vi "AbortAllMovements.vi"(8 "error in (no error)":errorcluster, 11 "CS++Motor in":refnum<class "CS++Motor.lvclass">) -> (0 "error out":errorcluster, 3 "CS++Motor out":refnum<class "CS++Motor.lvclass">)   [LabVIEW 2015, in "CS++Motor.lvlib" / "CS++Motor.lvclass"]
doc: "Stops the movement of all axes immeadiately."
uses:
  CS++Motor.lvclass
  CS++Motor.lvclass/CS++Motor.ctl
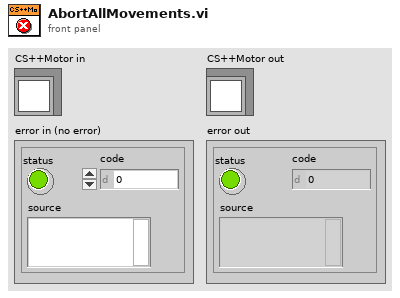
[diagram p1: front panel]
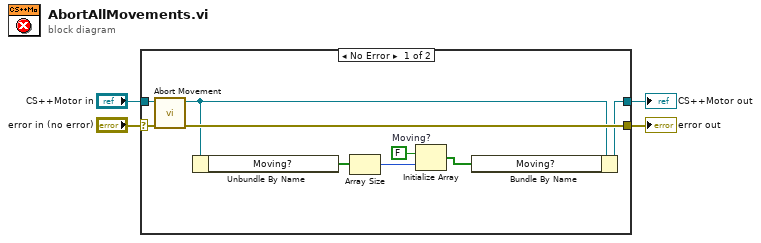
[diagram p0: block diagram]
diagram:
  n1 = case shown="No Error" "error in (no error)" {
    selector: "error in (no error)" -> [w12 w15]
    tunnel: [w11 w15] -> w3
    tunnel: [w10 w14] -> w4
    tunnel: "CS++Motor in" -> [w13 w14]
    frame No Error {
      w8 = FALSE  # Moving?
      n2 = call "Abort Movement.vi"("error in (no error)"=w12, "CS++Motor in"=w13) -> ("error out"=w11:errorcluster, "CS++Motor out"=w9:refnum<class "CS++Motor.lvclass">)  [unwired: 8 in]
      n3 = Unbundle By Name(w9) -> ("Moving?"=w6:bool[])
      n4 = Array Size(array=w6) -> (size(s)=w7:i32)
      n5 = Initialize Array(w8, w7) -> (w5:bool[])
      n6 = Bundle By Name(cluster=w9, "Moving?"=w5) -> (w10:refnum<class "CS++Motor.lvclass">)
    }
    frame Error {
    }
  }
  "error out" <- w3
  "CS++Motor out" <- w4
